vi "solar Ctrls Save.vi"(6 "ArrayDelimiters (1D,2D)":string[](array[string]), 7 "Section (\"\" = Use Target)":string, 8 "error in (no error)":errorcluster, 9 "Key Prefix (\"\")":string, 10 "Close Refnums? (T)":bool=TRUE, 11 "solar in":refnum<class "solar.lvclass">) -> (0 "error out":errorcluster, 2 "CtrlRefnums":refnum<vi>[](array[refnum]), 3 "solar out":refnum<class "solar.lvclass">)   [LabVIEW 2018]
doc: "This saves the registered control refnum values to the temporary configuration file (temporary.ini). Set Close Refnums? to true to close the control refnums."
uses:
  cfg/solar_cfg Write File (Ref).vi
  solar.lvclass
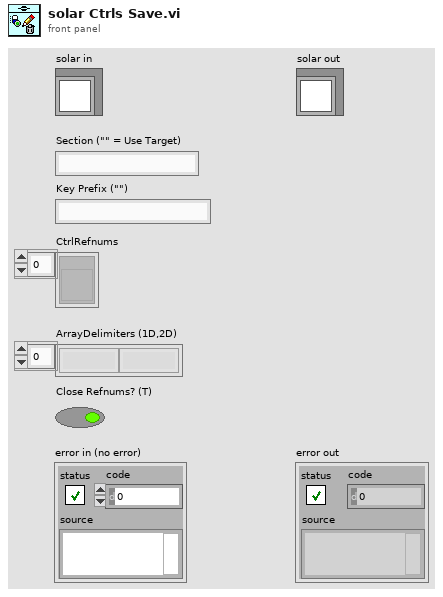
[diagram p1: front panel]
types:
  T1 = typedef "solar_app_ctl Info.ctl" = cluster{"AppName":string, "AppDir":path, "solar.ini":path, "ConfigsDir":path, "LogsDir":path, "CosmosDir":path, "ExePath":path, "vApp":string, "Part":string, "Setup":string, "Title":string, "Main.ini":path, "temp.ini":path, "vSOLAR":string, "Splash.png":string}
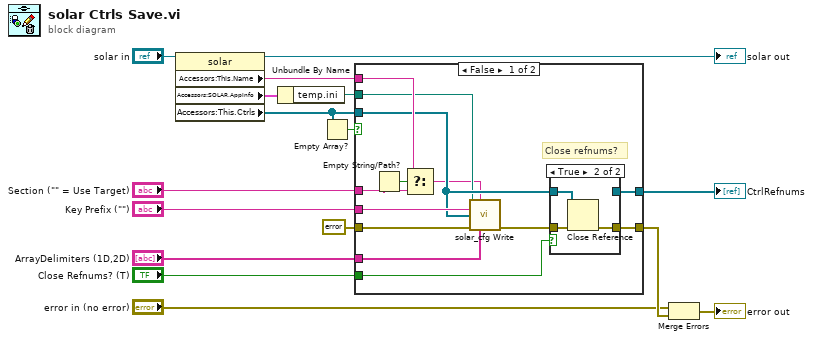
[diagram p0: block diagram]
diagram:
  n1 = property class="solar"(reference="solar in") -> (reference out=→"solar out":refnum<class "solar.lvclass">, "Accessors:This.Name"=w10:string, "Accessors:SOLAR.AppInfo"=w8:T1, "Accessors:This.Ctrls"=w4:refnum<vi>[])  [unwired: 1 in, 1 out]
  n2 = Unbundle By Name(w8) -> ("temp.ini"=w12:path)
  n3 = Empty Array?(array=w4) -> (empty?=w14:bool)
  n4 = case shown="False" w14 {
    tunnel: errorcluster {"status"=FALSE, "code"=0, "source"=""} ("error in (no error)") -> [w29 w36]
    tunnel: [w23 w36] -> w5
    tunnel: w4 -> [w19 w35]
    tunnel: "Key Prefix (\"\")" -> [w28 _]
    tunnel: w12 -> [w18 _]
    tunnel: "ArrayDelimiters (1D,2D)" -> [w20 _]
    tunnel: [w21 w35] -> w7
    tunnel: w10 -> [w26 _]
    tunnel: "Section (\"\" = Use Target)" -> [w25 _]
    tunnel: "Close Refnums? (T)" -> [w22 _]
    frame False {
      # "Close refnums?"
      n5 = Empty String/Path?(string/path=w25) -> (empty?=w27:bool)
      n6 = Select(t=w26, s=w27, f=w25) -> (s? t:f=w17:string)
      n7 = call-poly "solar_cfg Write.vi"("Config Path (*.ini)"=w18, "Section (\"\" = Use Filename)"=w17, "Key_Prefix (\"\")"=w28, "Ctrl Refnums"=w19, "error in (no error)"=w29, "ArrayDelimiters (1D,2D)"=w20) -> ("error out"=w24:errorcluster)  [unwired: 7 in, 2 out]
      n8 = case shown="True" w22 {
        tunnel: w24 -> [w30 w34]
        tunnel: [w30 w33] -> w23
        tunnel: w19 -> [w31 w32]
        tunnel: [w31 _] -> w21
        frame False {
        }
        frame True {
          n9 = Close Reference(reference=w32, error in (no error)=w34) -> (error out=w33:errorcluster)
        }
      }
    }
    frame True {
    }
  }
  "CtrlRefnums" <- w7
  n10 = Merge Errors("error in (no error)", w5) -> (→"error out":errorcluster)
